vi "tearDown.vi"(8 "error in (no error)":errorcluster, 11 "reference in":refnum<class "suite SSL Client.lvclass">) -> (0 "error out":errorcluster, 3 "reference out":refnum<class "suite SSL Client.lvclass">)   [LabVIEW 2013, in "suite SSL Client.lvclass"]
doc: "tearDown runs after the test method has completed. Use this method to clean up any operations or references that were opened by setUp or the test method. Unit tests should be independent of other unit tests so this VI should ensure that the next test can run in a 'clean' test environment."
uses:
  suite SSL Client.lvclass
  SSL_Lib/SSL-Context/SSL-Context.lvclass
  SSL_Lib/SSL-Lib/SSL-Lib.lvclass
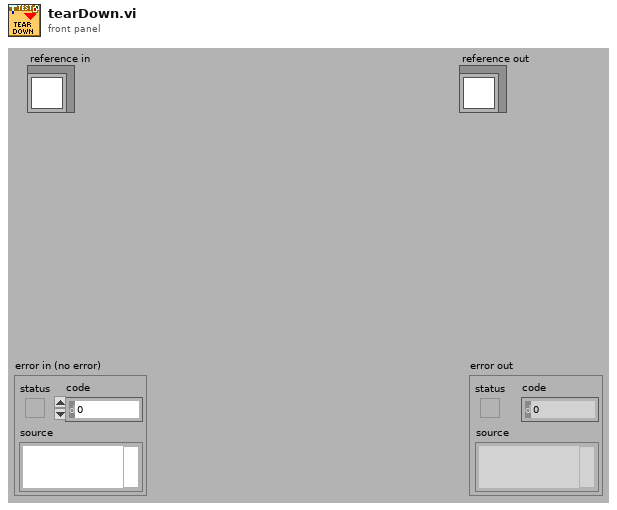
[diagram p1: front panel]
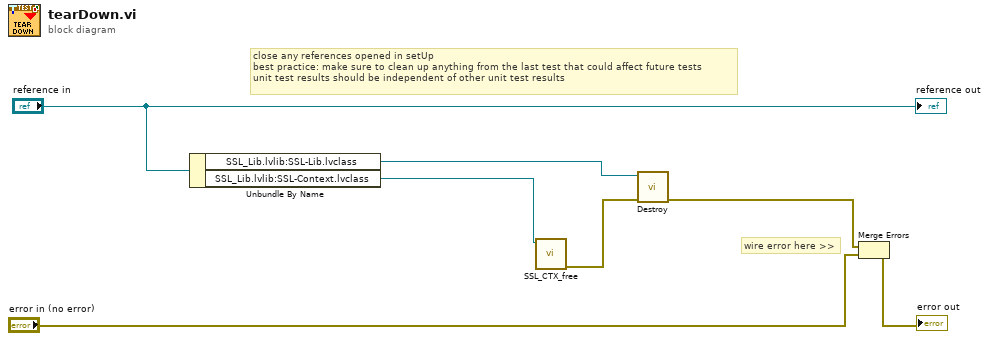
[diagram p0: block diagram]
diagram:
  # "wire error here >>"
  # "close any references opened in setUp\nbest practice: make sure to clean up anything from the last test that could affect future tests\nunit test results should be independent of other unit test results"
  n1 = Unbundle By Name("reference in") -> ("SSL_Lib.lvlib:SSL-Lib.lvclass"=w3:refnum<class "SSL-Lib.lvclass">, "SSL_Lib.lvlib:SSL-Context.lvclass"=w2:refnum<class "SSL-Context.lvclass">)
  n2 = call "SSL_CTX_free.vi"("SSL-Context in"=w2) -> ("error out"=w4:errorcluster)  [unwired: 10 in]
  n3 = call "Destroy.vi"("error in (no error)"=w4, "SSL-Lib in"=w3) -> ("error out"=w1:errorcluster)  [unwired: 9 in]
  n4 = Merge Errors(w1, "error in (no error)") -> (→"error out":errorcluster)
  "reference out" <- "reference in"
